vi "Assert 64 bit wired to 32 bit Type.vi"   [LabVIEW 2017]
uses:
  ae2a8e42-1705-40ca-9a85-37e96da610be.vi
  6698b199-9c51-4eeb-b7c8-706278b0f90a.vi
  39702413-5c4c-4f7d-848b-2e7116a58f57.vi
  589e4ee3-e11e-4dcc-b3fe-fad5ceb21069.vi
  db8402c5-9e09-4326-9251-2cdded9c337c.vi
  a3e51480-a4f9-474e-88e9-58ae78dca282.vi
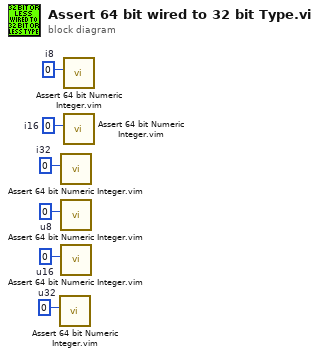
[diagram p0: block diagram]
diagram:
  w1 = u32 0  # u32
  w2 = u16 0  # u16
  w3 = u8 0  # u8
  w4 = 0  # i32
  w5 = i16 0  # i16
  w6 = i8 0  # i8
  n1 = call "Assert 64 bit Numeric Integer.vim"("Item in"=w1) -> ()  [unwired: 10 in, 1 out]
  n2 = call "Assert 64 bit Numeric Integer.vim"("Item in"=w4) -> ()  [unwired: 10 in, 1 out]
  n3 = call "Assert 64 bit Numeric Integer.vim"("Item in"=w3) -> ()  [unwired: 10 in, 1 out]
  n4 = call "Assert 64 bit Numeric Integer.vim"("Item in"=w2) -> ()  [unwired: 10 in, 1 out]
  n5 = call "Assert 64 bit Numeric Integer.vim"("Item in"=w6) -> ()  [unwired: 10 in, 1 out]
  n6 = call "Assert 64 bit Numeric Integer.vim"("Item in"=w5) -> ()  [unwired: 10 in, 1 out]
